vi "MCLB Request Edit Cell.vi"(8 "error in (no error)":errorcluster, 10 "Cell Position":T1, 11 "View in":refnum<class "MCListbox View.lvclass">) -> (0 "error out":errorcluster, 1 "Edited Cell":T1, 2 "Value":string, 3 "View out":refnum<class "MCListbox View.lvclass">, 5 "Modified?":bool)   [LabVIEW 2013, in "SET Project Editor.lvlib" / "MCListbox View.lvclass"]
uses:
  MCListbox View.lvclass
  <vilib>/Utility/miscctls.llb/LVRowAndColumnTypeDef.ctl
  MCListbox View.lvclass/MCListbox View.ctl
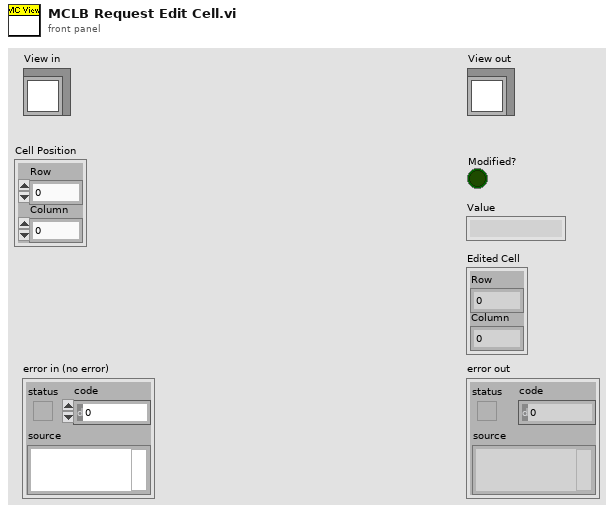
[diagram p1: front panel]
types:
  T1 = typedef "LVRowAndColumnTypeDef.ctl" = cluster{"Row":i32, "Column":i32}
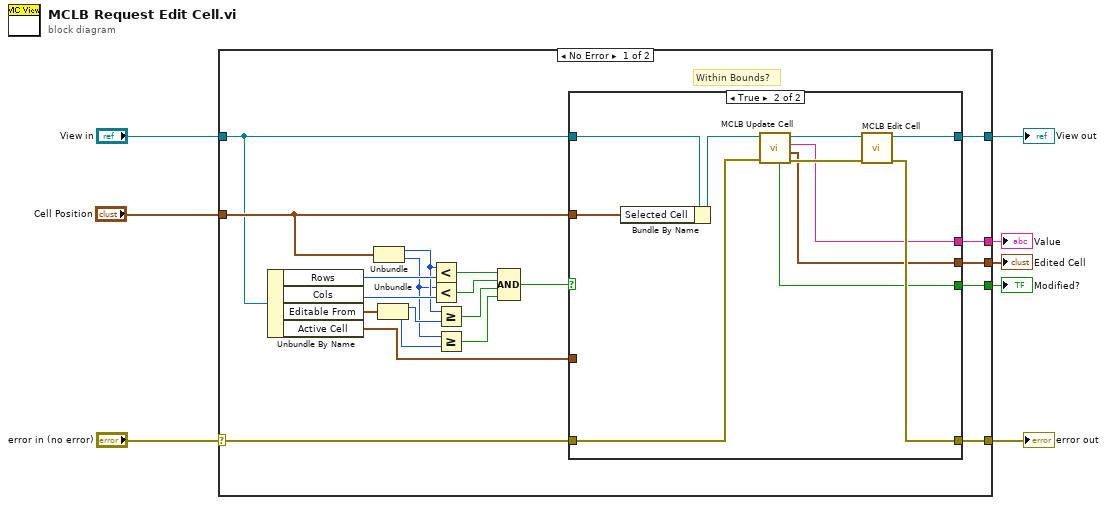
[diagram p0: block diagram]
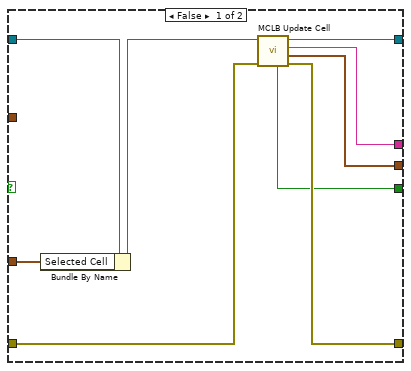
[diagram p2: hidden frame]
diagram:
  n1 = case shown="No Error" "error in (no error)" {
    selector: "error in (no error)" -> [w23 w51]
    tunnel: [w22 w51] -> w7
    tunnel: [w20 w50] -> w5
    tunnel: "View in" -> [w21 w50]
    tunnel: "Cell Position" -> [w24 _]
    tunnel: [w19 _] -> w1
    tunnel: [w18 _] -> w3
    tunnel: [w17 _] -> w2
    frame No Error {
      # "Within Bounds?"
      n2 = Unbundle By Name(w21) -> ("Rows"=w27:i32, "Cols"=w26:i32, "Editable From"=w14:T1, "Active Cell"=w15:T1)
      n3 = Unbundle(w24) -> ("Row"=w16:i32, "Column"=w11:i32)
      n4 = Unbundle(w14) -> ("Row"=w13:i32, "Column"=w12:i32)
      n5 = Less?(x=w16, y=w27) -> (x < y?=w29:bool)
      n6 = Less?(x=w11, y=w26) -> (x < y?=w28:bool)
      n7 = Greater Or Equal?(x=w16, y=w13) -> (x >= y?=w10:bool)
      n8 = Greater Or Equal?(x=w11, y=w12) -> (x >= y?=w9:bool)
      n9 = Compound Arithmetic op=AND(w29, w28, w10, w9) -> (w25:bool)
      n10 = case shown="True" w25 {
        tunnel: w24 -> [_ w49]
        tunnel: w15 -> [w35 _]
        tunnel: w21 -> [w37 w47]
        tunnel: w23 -> [w38 w45]
        tunnel: [w33 w44] -> w22
        tunnel: [w34 w48] -> w20
        tunnel: [w32 w41] -> w19
        tunnel: [w31 w40] -> w18
        tunnel: [w30 w39] -> w17
        frame False {
          n11 = Bundle By Name(cluster=w37, "Selected Cell"=w35) -> (w36:refnum<class "MCListbox View.lvclass">)
          n12 = call "MCLB Update Cell.vi"("error in (no error)"=w38, "View in"=w36) -> ("error out"=w33:errorcluster, "Active Cell"=w30:T1, "Value"=w31:string, "View out"=w34:refnum<class "MCListbox View.lvclass">, "Update?"=w32:bool)  [unwired: 5 in]
        }
        frame True {
          n13 = Bundle By Name(cluster=w47, "Selected Cell"=w49) -> (w46:refnum<class "MCListbox View.lvclass">)
          n14 = call "MCLB Update Cell.vi"("error in (no error)"=w45, "View in"=w46) -> ("error out"=w42:errorcluster, "Active Cell"=w39:T1, "Value"=w40:string, "View out"=w43:refnum<class "MCListbox View.lvclass">, "Update?"=w41:bool)  [unwired: 5 in]
          n15 = call "MCLB Edit Cell.vi"("error in (no error)"=w42, "View in"=w43) -> ("error out"=w44:errorcluster, "View out"=w48:refnum<class "MCListbox View.lvclass">)  [unwired: 8 in]
        }
      }
    }
    frame Error {
    }
  }
  "error out" <- w7
  "View out" <- w5
  "Value" <- w3
  "Edited Cell" <- w2
  "Modified?" <- w1
